vi "FF_readdress_devices.vi"(8 "error in (no error)":errorcluster, 9 "deviceID list":string[](array[string]), 10 "address list":string[](array[string]), 11 "refnum in":cluster{"Handle1":u32, "Handle2":u32}) -> (0 "Error Out":errorcluster, 1 "deviceID list out":string[](array[string]), 2 "device address list out":i32[](array[numeric]), 3 "refnum out":cluster{"Handle1":u32, "Handle2":u32})   [LabVIEW 2012]
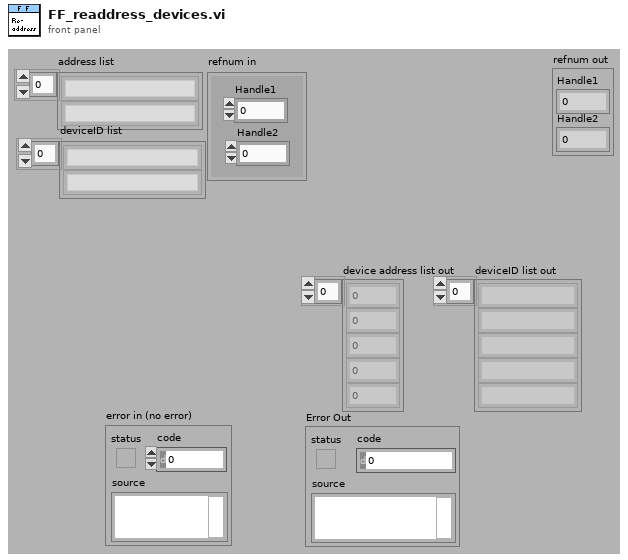
[diagram p1: front panel]
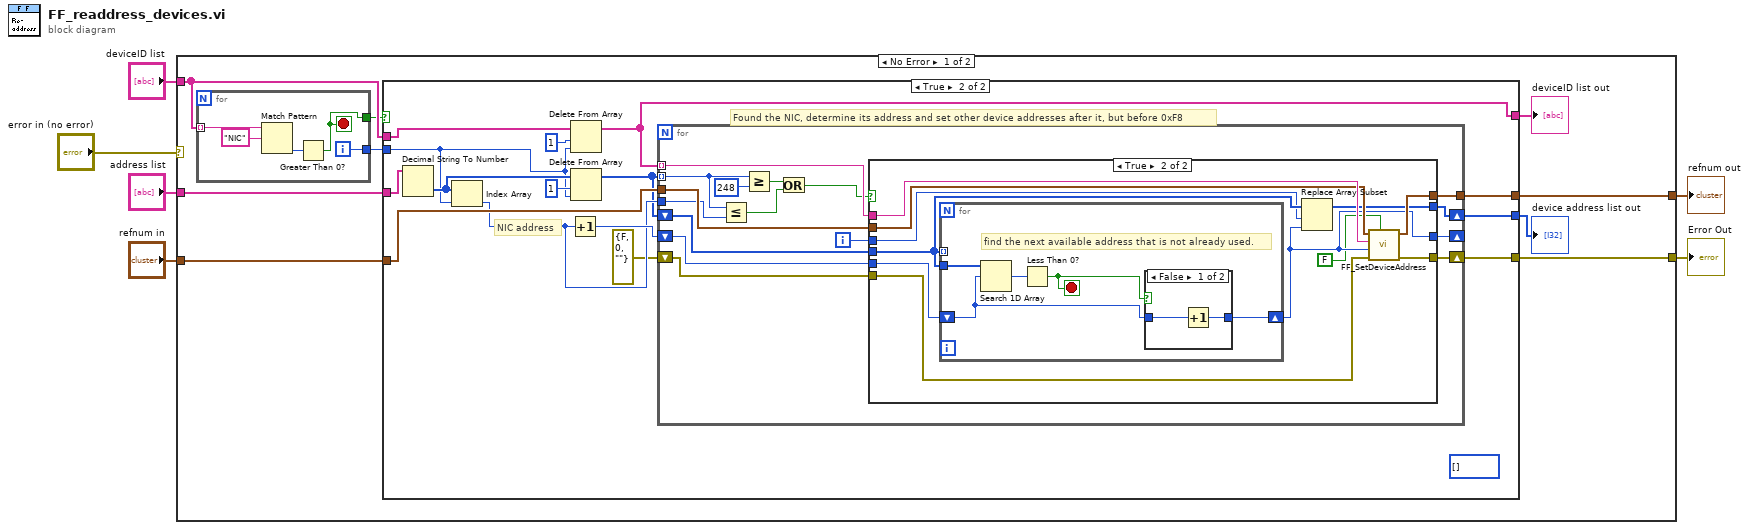
[diagram p0: block diagram]
diagram:
  n1 = case shown="No Error" "error in (no error)" {
    selector: "error in (no error)" -> [_ w77]
    tunnel: "refnum in" -> [w14 w76]
    tunnel: "deviceID list" -> [w11 _]
    tunnel: "address list" -> [w10 _]
    tunnel: [w8 w77] -> w6
    tunnel: [w7 w76] -> w1
    frame No Error {
      n2 = for {
        tunnel: w11 -> [w75] mode=indexing
        tunnel: [w72] -> w9
        tunnel: [w71] -> w15
        i -> [w71]
        stop <- w72 stop-if-true
        n3 = Match Pattern(string=w75, regular expression="NIC") -> (offset past match=w73:i32)  [unwired: 1 in, 3 out]
        n4 = Greater Than 0?(x=w73) -> (x > 0?=w72:bool)
      }
      n5 = case shown="True" w9 {
        tunnel: w15 -> [_ w23]
        tunnel: w10 -> [_ w25]
        tunnel: w14 -> [w16 w31]
        tunnel: [w16 w30] -> w7
        tunnel: w11 -> [_ w22]
        tunnel: [_ w21] -> w13
        tunnel: [_ w20] -> w12
        tunnel: [_ w19] -> w8
        frame False {
        }
        frame True {
          (unwired) i32[] []
          # "NIC address"
          # "Found the NIC, determine its address and set other device addresses after it, but before 0xF8"
          n6 = Decimal String To Number(string=w25) -> (number=w27:i32[])  [unwired: 2 in, 1 out]
          n7 = Index Array(array=w27, index=w23) -> (element=w28:i32)
          n8 = Increment(x=w28) -> (x+1=w29:i32)
          n9 = Delete From Array(array=w22, length=1, index=w23) -> (array with subset deleted=w20:string[])  [unwired: 1 out]
          n10 = Delete From Array(array=w27, length=1, index=w23) -> (array with subset deleted=w17:i32[])  [unwired: 1 out]
          n11 = for {
            tunnel: w20 -> [w46] mode=indexing
            tunnel: w31 -> [w45]
            tunnel: [w44] -> w30
            tunnel: w17 -> [w43] mode=indexing
            tunnel: w28 -> [w39]
            shift-right: [w36] -> _
            shift-left: w29 -> [w37]
            shift-right: [w34] -> w21
            shift-left: w17 -> [w38]
            shift-right: [w33] -> w19
            shift-left: errorcluster {"status"=FALSE, "code"=0, "source"=""} ("error out") -> [w32]
            i -> [w35]
            n12 = Less Or Equal?(x=w43, y=w39) -> (x <= y?=w41:bool)
            n13 = Greater Or Equal?(x=w43, y=248) -> (x >= y?=w40:bool)
            n14 = Or(x=w40, y=w41) -> (x .or. y?=w42:bool)
            n15 = case shown="True" w42 {
              tunnel: w46 -> [_ w62]
              tunnel: w45 -> [w51 w61]
              tunnel: [w51 w60] -> w44
              tunnel: w38 -> [w49 w57]
              tunnel: w37 -> [w50 w59]
              tunnel: [w50 w58] -> w36
              tunnel: w35 -> [_ w56]
              tunnel: [w49 w55] -> w34
              tunnel: [w48 w54] -> w33
              tunnel: w32 -> [w48 w53]
              frame False {
              }
              frame True {
                n16 = for {
                  tunnel: w57 -> [w67]
                  shift-right: [w63] -> w58
                  shift-left: w59 -> [w64]
                  tunnel: w57 -> [_] mode=indexing
                  stop <- w65 stop-if-true
                  # "find the next available address that is not already used."
                  n17 = Search 1D Array(1D array=w67, element=w64) -> (index of element=w66:i32)  [unwired: 1 in]
                  n18 = Less Than 0?(x=w66) -> (x < 0?=w65:bool)
                  n19 = case shown="False" w65 {
                    tunnel: w64 -> [w69 w70]
                    tunnel: [w68 w70] -> w63
                    frame False {
                      n20 = Increment(x=w69) -> (x+1=w68:i32)
                    }
                    frame True {
                    }
                  }
                }
                n21 = Replace Array Subset(array=w57, new element=w58, index=w56) -> (w55:i32[])
                n22 = call "FF_SetDeviceAddress.vi"("Is pdTag"=FALSE, "error in (no error)"=w53, "address"=w58, "pdTag/deviceID"=w62, "refnum in"=w61) -> ("error out"=w54:errorcluster, "refnum out"=w60:cluster{"Handle1":u32, "Handle2":u32})  [unwired: 5 in]
              }
            }
          }
        }
      }
      "device address list out" <- w13
      "deviceID list out" <- w12
    }
    frame Error {
    }
  }
  "Error Out" <- w6
  "refnum out" <- w1
